vi "Create.vi"(7 "selection_dropdown in":refnum<class "selection_dropdown.lvclass">, 8 "error in (no error)":errorcluster, 11 "ref":refnum<vi>) -> (0 "error out":errorcluster, 3 "selection_dropdown out":refnum<class "selection_dropdown.lvclass">)   [LabVIEW 2024, in "selection_dropdown.lvclass"]
uses:
  selection_dropdown.lvclass
  selection_dropdown.lvclass/selection_dropdown.ctl
  Typedefs/Selection Dropdown.ctl
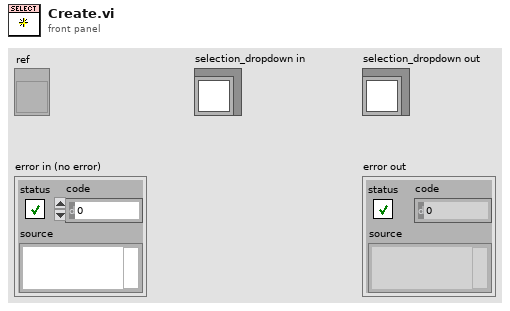
[diagram p1: front panel]
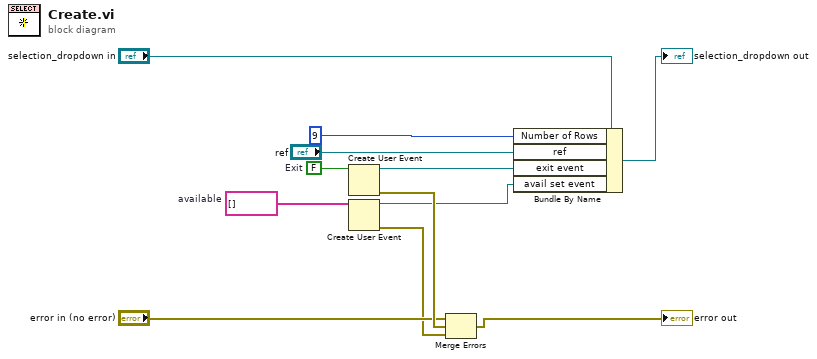
[diagram p0: block diagram]
diagram:
  w3 = string[] []  # available
  w10 = FALSE  # Exit
  n1 = Create User Event(user event datatype=w10) -> (user event=w9:refnum<user-event>, error out=w7:errorcluster)  [unwired: 1 in]
  n2 = Create User Event(user event datatype=w3) -> (user event=w1:refnum<user-event>, error out=w2:errorcluster)  [unwired: 1 in]
  n3 = Merge Errors("error in (no error)", w7, w2) -> (→"error out":errorcluster)
  n4 = Bundle By Name(cluster="selection_dropdown in", "Number of Rows"=u32 9, "ref"="ref", "exit event"=w9, "avail set event"=w1) -> (→"selection_dropdown out":refnum<class "selection_dropdown.lvclass">)
